vi "Read VIRef.vi"(8 "error in (no error)":errorcluster, 11 "CtlReferences in":refnum<class "CtlReferences.lvclass">) -> (0 "error out":errorcluster, 2 "VIRef":refnum<vi>, 3 "CtlReferences out":refnum<class "CtlReferences.lvclass">)   [LabVIEW 2020, in "CtlReferences.lvlib" / "CtlReferences.lvclass"]
uses:
  CtlReferences.lvclass
  CtlReferences.lvclass/CtlReferences.ctl
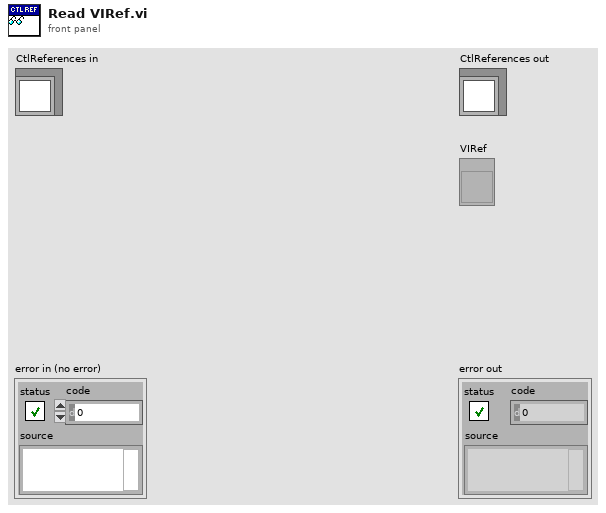
[diagram p1: front panel]
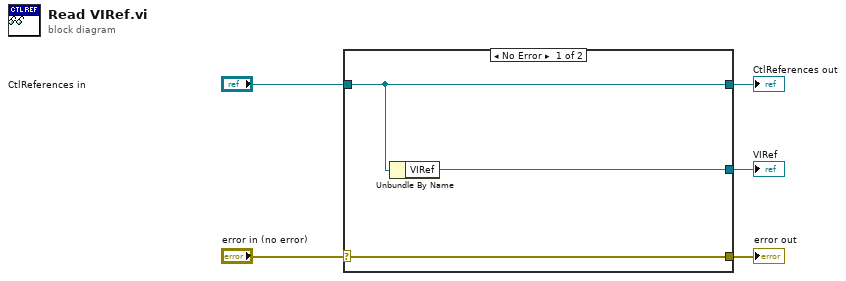
[diagram p0: block diagram]
diagram:
  n1 = case shown="No Error" "error in (no error)" {
    selector: "error in (no error)" -> [w8 w9]
    tunnel: [w8 w9] -> w4
    tunnel: [w7 w10] -> w2
    tunnel: "CtlReferences in" -> [w7 w10]
    tunnel: [w6 _] -> w1
    frame No Error {
      n2 = Unbundle By Name(w7) -> ("VIRef"=w6:refnum<vi>)
    }
    frame Error {
    }
  }
  "error out" <- w4
  "CtlReferences out" <- w2
  "VIRef" <- w1
